vi "Command.Diagnostic Data Lookup Table Action.vi"(6 "command":T2, 7 "Name":string, 8 "error in (no error)":errorcluster, 9 "Signals":dbl[](array[numeric]), 10 "Signal In":dbl, 11 "Diag Data Ref":T1) -> (0 "error out":errorcluster {"code" min=0 max=0}, 1 "Signals Out":dbl[](array[numeric]), 2 "Signal Out":dbl, 3 "Diag Data Ref out":T1)   [LabVIEW 2015, in "J1939 Addon Engine.lvlib"]
uses:
  J1939 Addon Engine.lvlib
  Types/Command.Diagnostic Data Lookup Table Reference.ctl
  Types/Command.Diagnostic Data Lookup Table State Variables.ctl
  Types/Command.Diagnostic Data Lookup Table Action.ctl
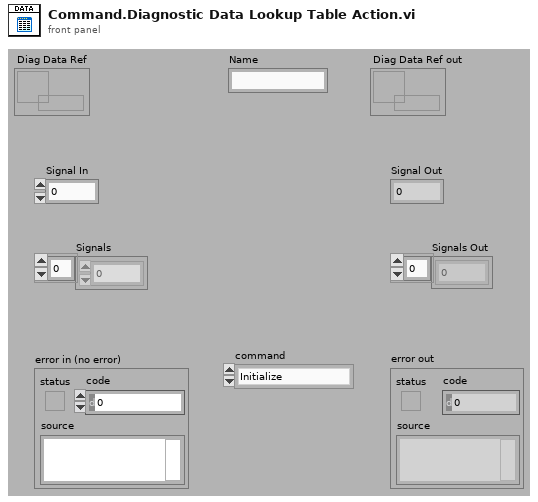
[diagram p1: front panel]
types:
  T1 = typedef "J1939 Addon Engine.lvlib/Command.Diagnostic Data Lookup Table Reference.ctl" = refnum<data-value>
  T2 = typedef "J1939 Addon Engine.lvlib/Command.Diagnostic Data Lookup Table Action.ctl" = enum16{"Initialize", "Get All", "Set All", "Set Value", "Get Value"}
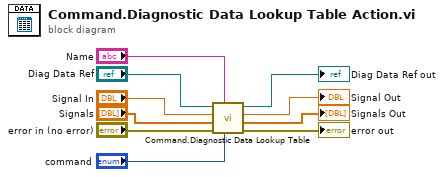
[diagram p0: block diagram]
diagram:
  n1 = call "Command.Diagnostic Data Lookup Table.vi"("command"="command", "Name"="Name", "error in (no error)"="error in (no error)", "Signals"="Signals", "Signal In"="Signal In", "Diag Data Ref"="Diag Data Ref") -> ("error out"=→"error out":errorcluster, "Signals Out"=→"Signals Out":dbl[], "Signal Out"=→"Signal Out":dbl, "Diag Data Ref out"=→"Diag Data Ref out":T1)  [unwired: 2 in]
